vi "WriteSpectrograms.vi"(4 "Array":i8[][][](array[numeric]), 6 "Doppler Params":T1={"Dopp Filter Order"=0, "Window length"=0, "Window Increment"=0, "Start f"=0.05, "lDoppler cutouff"=0.0, "FFT Length"=512, "SlowTime (Hz)"=100.0} {"Start f" format="%0.3f"; "SlowTime (Hz)" format="%0.1f"; "lDoppler cutouff" format="%0.3f"}, 8 "row #":i32, 9 "Slow Time Pt Mark":i32, 10 "Total length":i32, 11 "Byte Stream File in":string="test") -> ()   [LabVIEW 2022 SP3]
uses:
  DopplerParams.ctl
panel:
  out "size(s)":i32[](array[numeric])
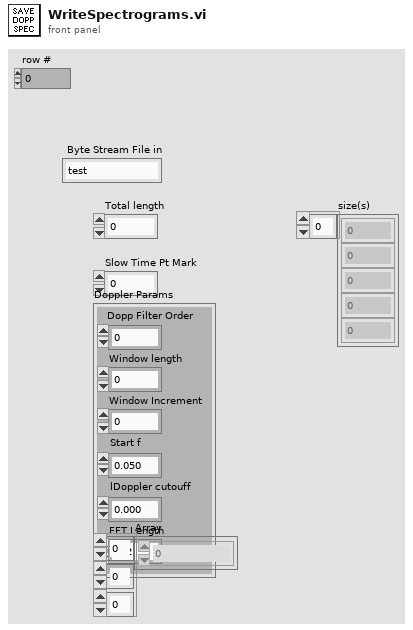
[diagram p1: front panel]
types:
  T1 = typedef "DopplerParams.ctl" = cluster{"Dopp Filter Order":i32, "Window length":i32, "Window Increment":i32, "Start f":dbl, "lDoppler cutouff":dbl, "FFT Length":i32, "SlowTime (Hz)":dbl}
  T2 = enum16{"big-endian, network order", "native, host order", "little-endian"}
  T3 = enum16{"open", "replace", "create", "open or create", "replace or create", "replace or create with confirmation"}
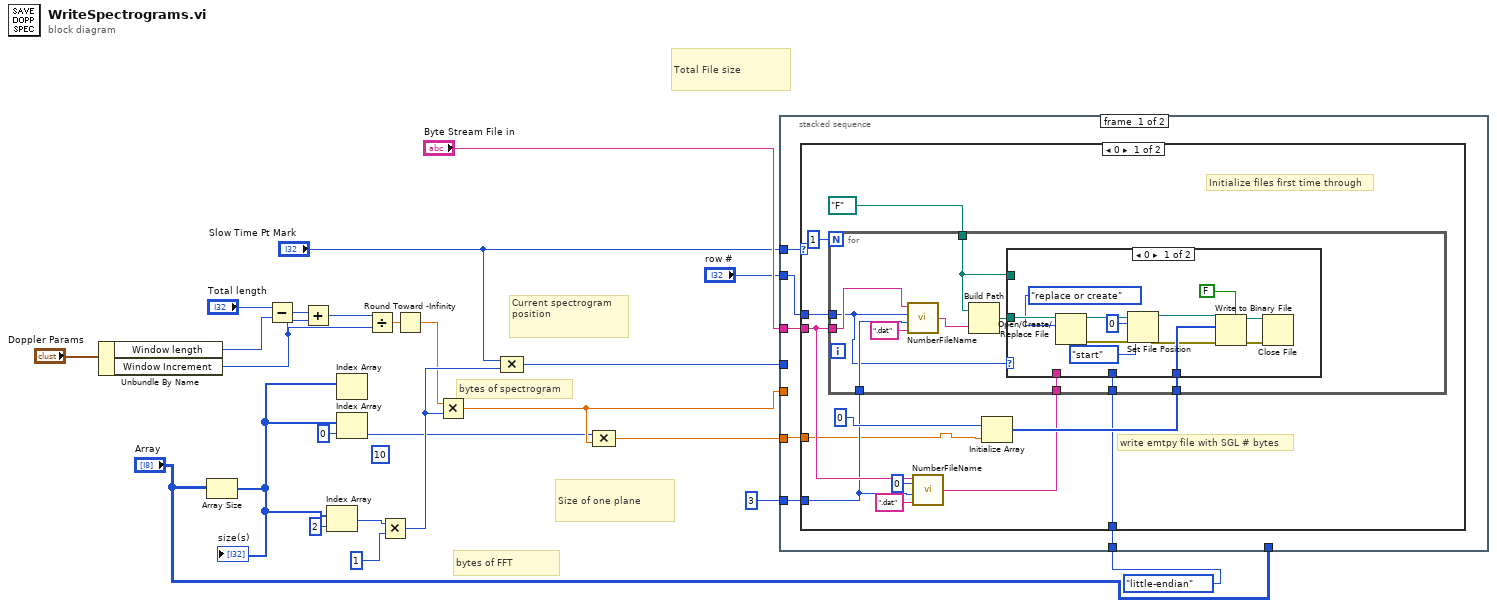
[diagram p0: block diagram]
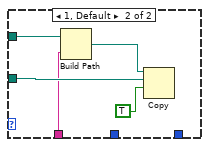
[diagram p2: hidden frame]
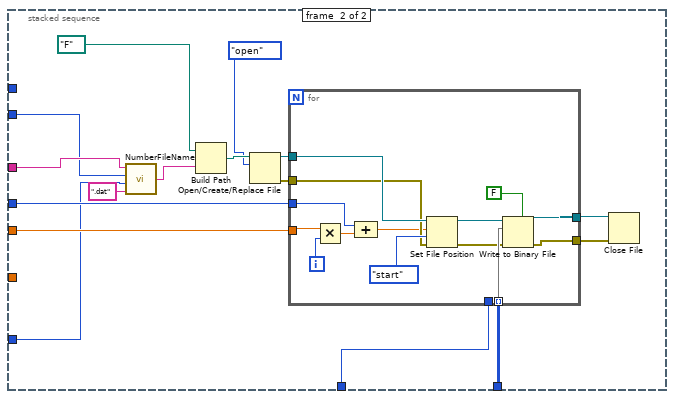
[diagram p4: hidden frame]
diagram:
  (unwired) 10 ("element")
  # "Total File size"
  # "Size of one plane"
  # "Current spectrogram position"
  # "bytes of FFT"
  # "bytes of spectrogram"
  n1 = Unbundle By Name("Doppler Params") -> ("Window length"=w19:i32, "Window Increment"=w20:i32)
  n2 = Array Size(array="Array") -> (size(s)=w23:i32[])
  "size(s)" <- w23
  n3 = Subtract(x="Total length", y=w19) -> (x-y=w15:i32)
  n4 = Add(x=w15, y=w20) -> (x+y=w14:i32)
  n5 = Index Array(array=w23, index=2) -> (element=w13:i32)
  n6 = Index Array(array=w23) -> ()  [unwired: 1 in, 1 out]
  n7 = Index Array(array=w23, index=0) -> (element=w5:i32)
  n8 = Divide(x=w14, y=w20) -> (x/y=w16:dbl)
  n9 = Multiply(x=w13, y=1) -> (x*y=w11:i32)
  n10 = Round Toward -Infinity(1:w16) -> (0:w10:dbl)
  n11 = Multiply(x=w10, y=w11) -> (x*y=w9:dbl)
  n12 = Compound Arithmetic op=MULTIPLY("Slow Time Pt Mark", w11) -> (w24:i32)
  n13 = Compound Arithmetic op=MULTIPLY(w5, w9) -> (w8:dbl)
  n14 = stacked-sequence {
    tunnel: w24 -> [_ w85]
    tunnel: "Array" -> [_ w84]
    tunnel: w9 -> [_ w83]
    tunnel: w8 -> [w30 _]
    tunnel: "Byte Stream File in" -> [w29 w82]
    tunnel: "Slow Time Pt Mark" -> [w28 _]
    tunnel: i16 3 ("d") -> [w27 w80]
    tunnel: "row #" -> [w26 w74]
    tunnel: T2."little-endian" ("byte order (0:big-endian, network order)") -> [w25 w71]
    frame #0 {
      n15 = case shown="0" w28 {
        tunnel: w30 -> [w32 _]
        tunnel: w29 -> [w39 _]
        tunnel: w27 -> [w35 _]
        tunnel: w26 -> [w34 _]
        tunnel: w25 -> [w31 _]
        frame 0 {
          # "write emtpy file with SGL # bytes"
          # "Initialize files first time through"
          n16 = call "NumberFileName.vi"("String"=".dat", "Digits"=w35, "File number"=0, "file name"=w39) -> ("Numbered File"=w38:string)
          n17 = Initialize Array(i8 0, w32) -> (w40:i8[])
          n18 = for {
            N: 1 -> [_]
            tunnel: w39 -> [w47]
            tunnel: path "F:/" ("base path") -> [w49]
            tunnel: w40 -> [w51]
            tunnel: w38 -> [w50]
            tunnel: w35 -> [w45]
            tunnel: w34 -> [w44]
            tunnel: w31 -> [w43]
            n19 = call "NumberFileName.vi"("String"=".dat", "Digits"=w45, "File number"=w44, "file name"=w47) -> ("Numbered File"=w46:string)
            n20 = Build Path(base path=w49, name or relative path=w46) -> (appended path=w52:path)
            n21 = case shown="0" w44 {
              tunnel: w52 -> [w64 w68]
              tunnel: w51 -> [w63 _]
              tunnel: w50 -> [_ w67]
              tunnel: w49 -> [_ w66]
              tunnel: w43 -> [_ _]
              frame 0 {
                n22 = Open/Create/Replace File(file path (use dialog)=w64, operation (0:open)=T3."replace or create") -> (refnum out=w57:refnum<file>, error out=w58:errorcluster)  [unwired: 4 in, 1 out]
                n23 = Set File Position(offset (in bytes) (0)=i64 0, refnum=w57, from (0:start)=enum16{"start", "end", "current"}."start", error in=w58) -> (refnum out=w56:refnum<file>, error out=w55:errorcluster)
                n24 = Write to Binary File(file (use dialog)=w56, data=w63, error in=w55, 5:FALSE ("prepend array or string size? (T)")) -> (refnum out=w61:refnum<file>, error out=w59:errorcluster)  [unwired: 2 in, 1 out]
                n25 = Close File(refnum=w61, error in=w59) -> ()  [unwired: 2 out]
              }
              frame 1, Default {
                n26 = Build Path(base path=w66, name or relative path=w67) -> (appended path=w65:path)
                n27 = Copy(9:TRUE ("overwrite (F)"), 10:w68, 11:w65) -> ()  [unwired: 2 in, 3 out]
              }
            }
          }
        }
        frame 1, Default {
        }
      }
    }
    frame #1 {
      n28 = call "NumberFileName.vi"("String"=".dat", "Digits"=w80, "File number"=w74, "file name"=w82) -> ("Numbered File"=w75:string)
      n29 = Build Path(base path=path "F:/", name or relative path=w75) -> (appended path=w79:path)
      n30 = Open/Create/Replace File(file path (use dialog)=w79, operation (0:open)=T3."open") -> (refnum out=w77:refnum<file>, error out=w73:errorcluster)  [unwired: 4 in, 1 out]
      n31 = for {
        tunnel: w84 -> [w98] mode=indexing
        tunnel: [w99] -> w78
        tunnel: w83 -> [w96]
        tunnel: w85 -> [w94]
        tunnel: w77 -> [w93]
        tunnel: w73 -> [w90]
        tunnel: [w89] -> w72
        tunnel: w71 -> [_]
        i -> [w97]
        n32 = Multiply(x=w96, y=w97) -> (x*y=w95:dbl)
        n33 = Compound Arithmetic op=ADD(w94, w95) -> (w87:dbl)
        n34 = Set File Position(offset (in bytes) (0)=w87, refnum=w93, from (0:start)=enum16{"start", "end", "current"}."start", error in=w90) -> (refnum out=w88:refnum<file>, error out=w91:errorcluster)
        n35 = Write to Binary File(file (use dialog)=w88, data=w98, error in=w91, 5:FALSE ("prepend array or string size? (T)")) -> (refnum out=w99:refnum<file>, error out=w89:errorcluster)  [unwired: 2 in, 1 out]
      }
      n36 = Close File(refnum=w78, error in=w72) -> ()  [unwired: 2 out]
    }
  }
